vi "Get Class Default Value.vi"(7 "error in (no error)":errorcluster, 10 "LabVIEW Object":refnum<class>) -> (0 "error out":errorcluster, 3 "Default Value of Class":refnum<class>)   [LabVIEW 2020, in "Utilities.lvlib"]
doc: "Gets the default value of the object's class."
uses:
  Utilities.lvlib
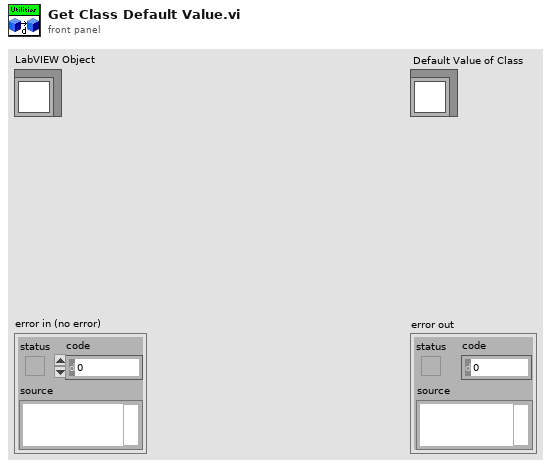
[diagram p1: front panel]
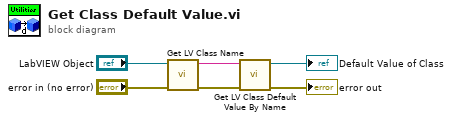
[diagram p0: block diagram]
diagram:
  n1 = call <vilib>:"Get LV Class Name.vi"("error in (no error)"="error in (no error)", "object"="LabVIEW Object") -> ("error out"=w5:errorcluster, "class name"=w4:string)  [unwired: 8 in]
  n2 = call <vilib>:"Get LV Class Default Value By Name.vi"("error in (no error)"=w5, "class name"=w4) -> ("error out"=→"error out":errorcluster, "object"=→"Default Value of Class":refnum<class>)  [unwired: 8 in]
